vi "Read Module Menu Name.vi"(8 "error in":errorcluster, 11 "Tag Bus Web Interface editor node in":refnum<class "Tag Bus Web Interface editor node.lvclass">) -> (0 "error out":errorcluster, 2 "Menu Name":string, 3 "Tag Bus Web Interface editor node out":refnum<class "Tag Bus Web Interface editor node.lvclass">)   [LabVIEW 2013, in "Tag Bus Web Interface editor node.lvclass"]
uses:
  Tag Bus Web Interface editor node.lvclass
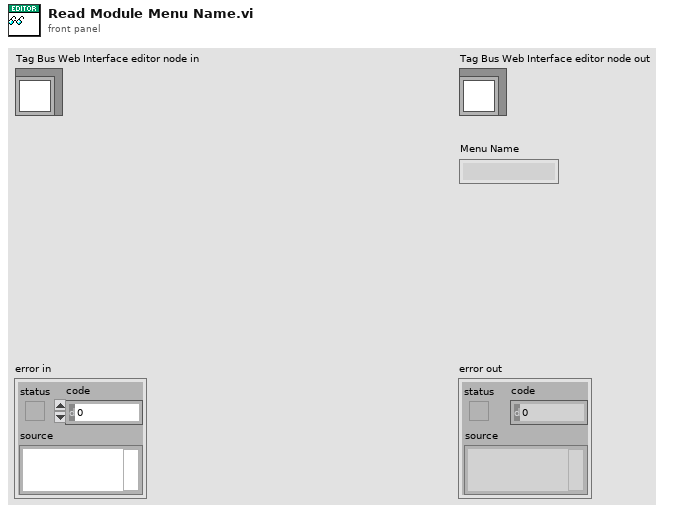
[diagram p1: front panel]
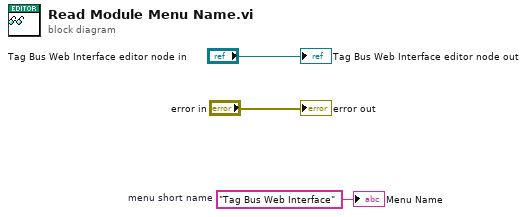
[diagram p0: block diagram]
diagram:
  w1 = "Tag Bus Web Interface"  # menu short name
  "error out" <- "error in"
  "Tag Bus Web Interface editor node out" <- "Tag Bus Web Interface editor node in"
  "Menu Name" <- w1
